vi "Call_Python.vi"() -> ()   [LabVIEW 2018]
panel:
  out "数值 2":u64
  out "返回值 2":u64
  in  "数值":u64
  in  "模块路径 2":path
  out "返回值":string
  in  "模块路径":path
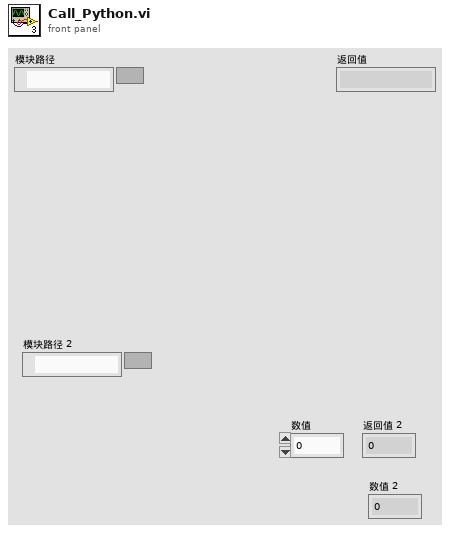
[diagram p1: front panel]
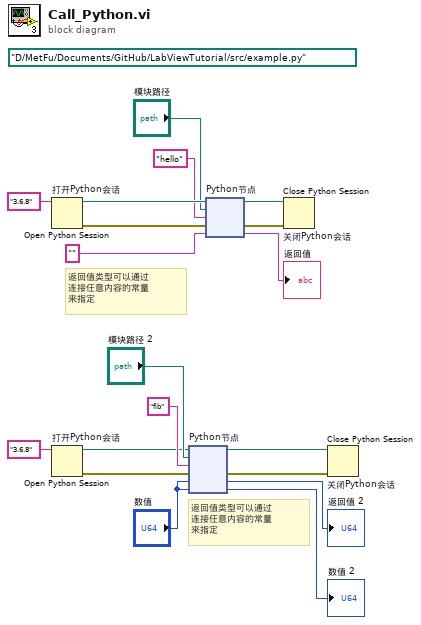
[diagram p0: block diagram]
diagram:
  (unwired) path "D:/MetFu/Documents/GitHub/LabViewTutorial/src/example.py" ("模块路径")
  # "返回值类型可以通过\n连接任意内容的常量\n来指定"
  # "返回值类型可以通过\n连接任意内容的常量\n来指定"
  n1 = Open Python Session "打开Python会话"(python version="3.6.8" ("Python版本")) -> (session out=w18:refnum<k35>, error out=w16:errorcluster)  [unwired: 2 in]
  n2 = Open Python Session "打开Python会话"(python version="3.6.8" ("Python版本")) -> (session out=w5:refnum<k35>, error out=w7:errorcluster)  [unwired: 2 in]
  n3 = node "Python节点"(w5, "模块路径 2", "fib" ("函数名称"), w7, "数值", "数值") -> (w6:refnum<k35>, w8:errorcluster, →"返回值 2":u64, →"数值 2":u64)  [unwired: 2 out]
  n4 = node "Python节点"(w18, "模块路径", "hello" ("函数名称"), w16, "") -> (w17:refnum<k35>, w15:errorcluster, →"返回值":string)  [unwired: 2 out]
  n5 = Close Python Session "关闭Python会话"(session in=w17, error in=w15) -> ()  [unwired: 1 out]
  n6 = Close Python Session "关闭Python会话"(session in=w6, error in=w8) -> ()  [unwired: 1 out]
